vi "TCtrlSeething.vi"() -> ()   [LabVIEW 2018]
uses:
  <vilib>/Utility/miscctls.llb/LVPointTypeDef.ctl
  <vilib>/Utility/error.llb/DialogType.ctl
panel:
  in  "基数可见":bool
  in  "增量可见":bool
  in  "标题可见":bool
  in  "标签可见":bool
  in  "数字精度":i32 min=0 max=8 step=1
  in  "显示格式":u16(ring) items=["十进制", "科学计数法", "工程计数", "二进制", "八进制", "十六进制", "相对时间", "时间和日期", "SI符号"]
  in  "字体格式":enum16{"正常", "粗体", "斜体", "删除线", "下划线"}(ring)
  in  "字体大小":i32
  in  "文本文字颜色":u32(colorbox)
  in  "文本前景色":u32(colorbox)
  in  "文本背景色":u32(colorbox)
  in  "控件前景色":u32(colorbox)
  in  "控件背景色":u32(colorbox)
  in  "数值":dbl
  in  "控件排布前面板.位置_前.位置":T1 caption="数字显示控件大小"
  in  "设定":bool
  out "Error Report":string
  out "Current State":string
  in  "Data Structure":T2
  in  "OK":bool
  in  "Exit Program":bool
  in  "Error":bool
  in  "Parameter":T3={"Q-HighLevel"="Q-HighLevel", "Q-Local"="Enginex", "Data"=variant}
  # "字体设置"
  # "示例"
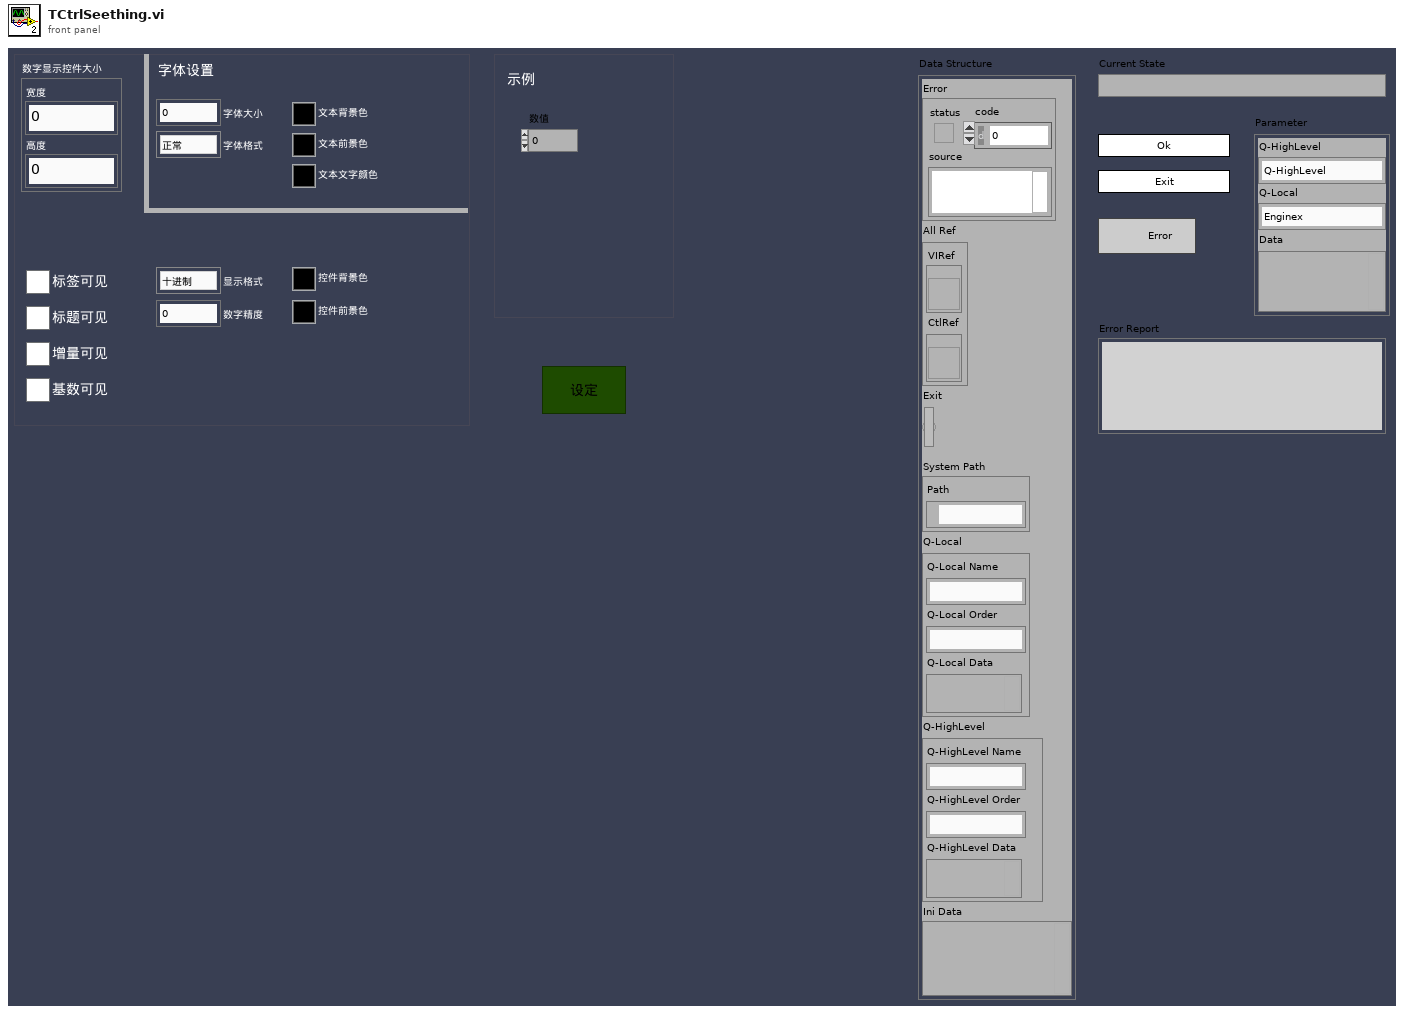
[diagram p1: front panel]
types:
  T1 = typedef "LVPointTypeDef.ctl" = cluster{"Horizontal":i16, "Vertical":i16}
  T2 = cluster{"Error":errorcluster, "All Ref":cluster{"VIRef":refnum<vi>, "CtlRef":refnum<vi>}, "Exit":bool, "System Path":cluster{"Path":path}, "Q-Local":cluster{"Q-Local Name":string, "Q-Local Order":string, "Q-Local Data":variant}, "Q-HighLevel":cluster{"Q-HighLevel Name":string, "Q-HighLevel Order":string, "Q-HighLevel Data":variant}, "Ini Data":variant}
  T3 = cluster{"Q-HighLevel":string, "Q-Local":string, "Data":variant}
  T4 = typedef "eventvkey.ctl" = enum16{"ASCII", "Enter", "Return", "Shift", "Ctrl", "Alt", "Cmd", "Opt", "Caps", "NumLock", "Clear", "Break", "Up", "Down", "Left", "Right", "Insert", "Delete", "Home", "End", "PageUp", "PageDown", "Escape", "Help", "Pause", "ScrollLock", "F1", "F2", "F3", "F4", "F5", "F6", "F7", "F8", "F9", "F10", "F11", "F12", "F13", "F14", "F15", "F16", "F17", "F18", "F19", "F20", "F21", "F22", "F23", "F24", "Play", "VolumeUp", "VolumeDown", "Mute", "Two Byte Char"}
  T5 = typedef "DialogType.ctl" = u16
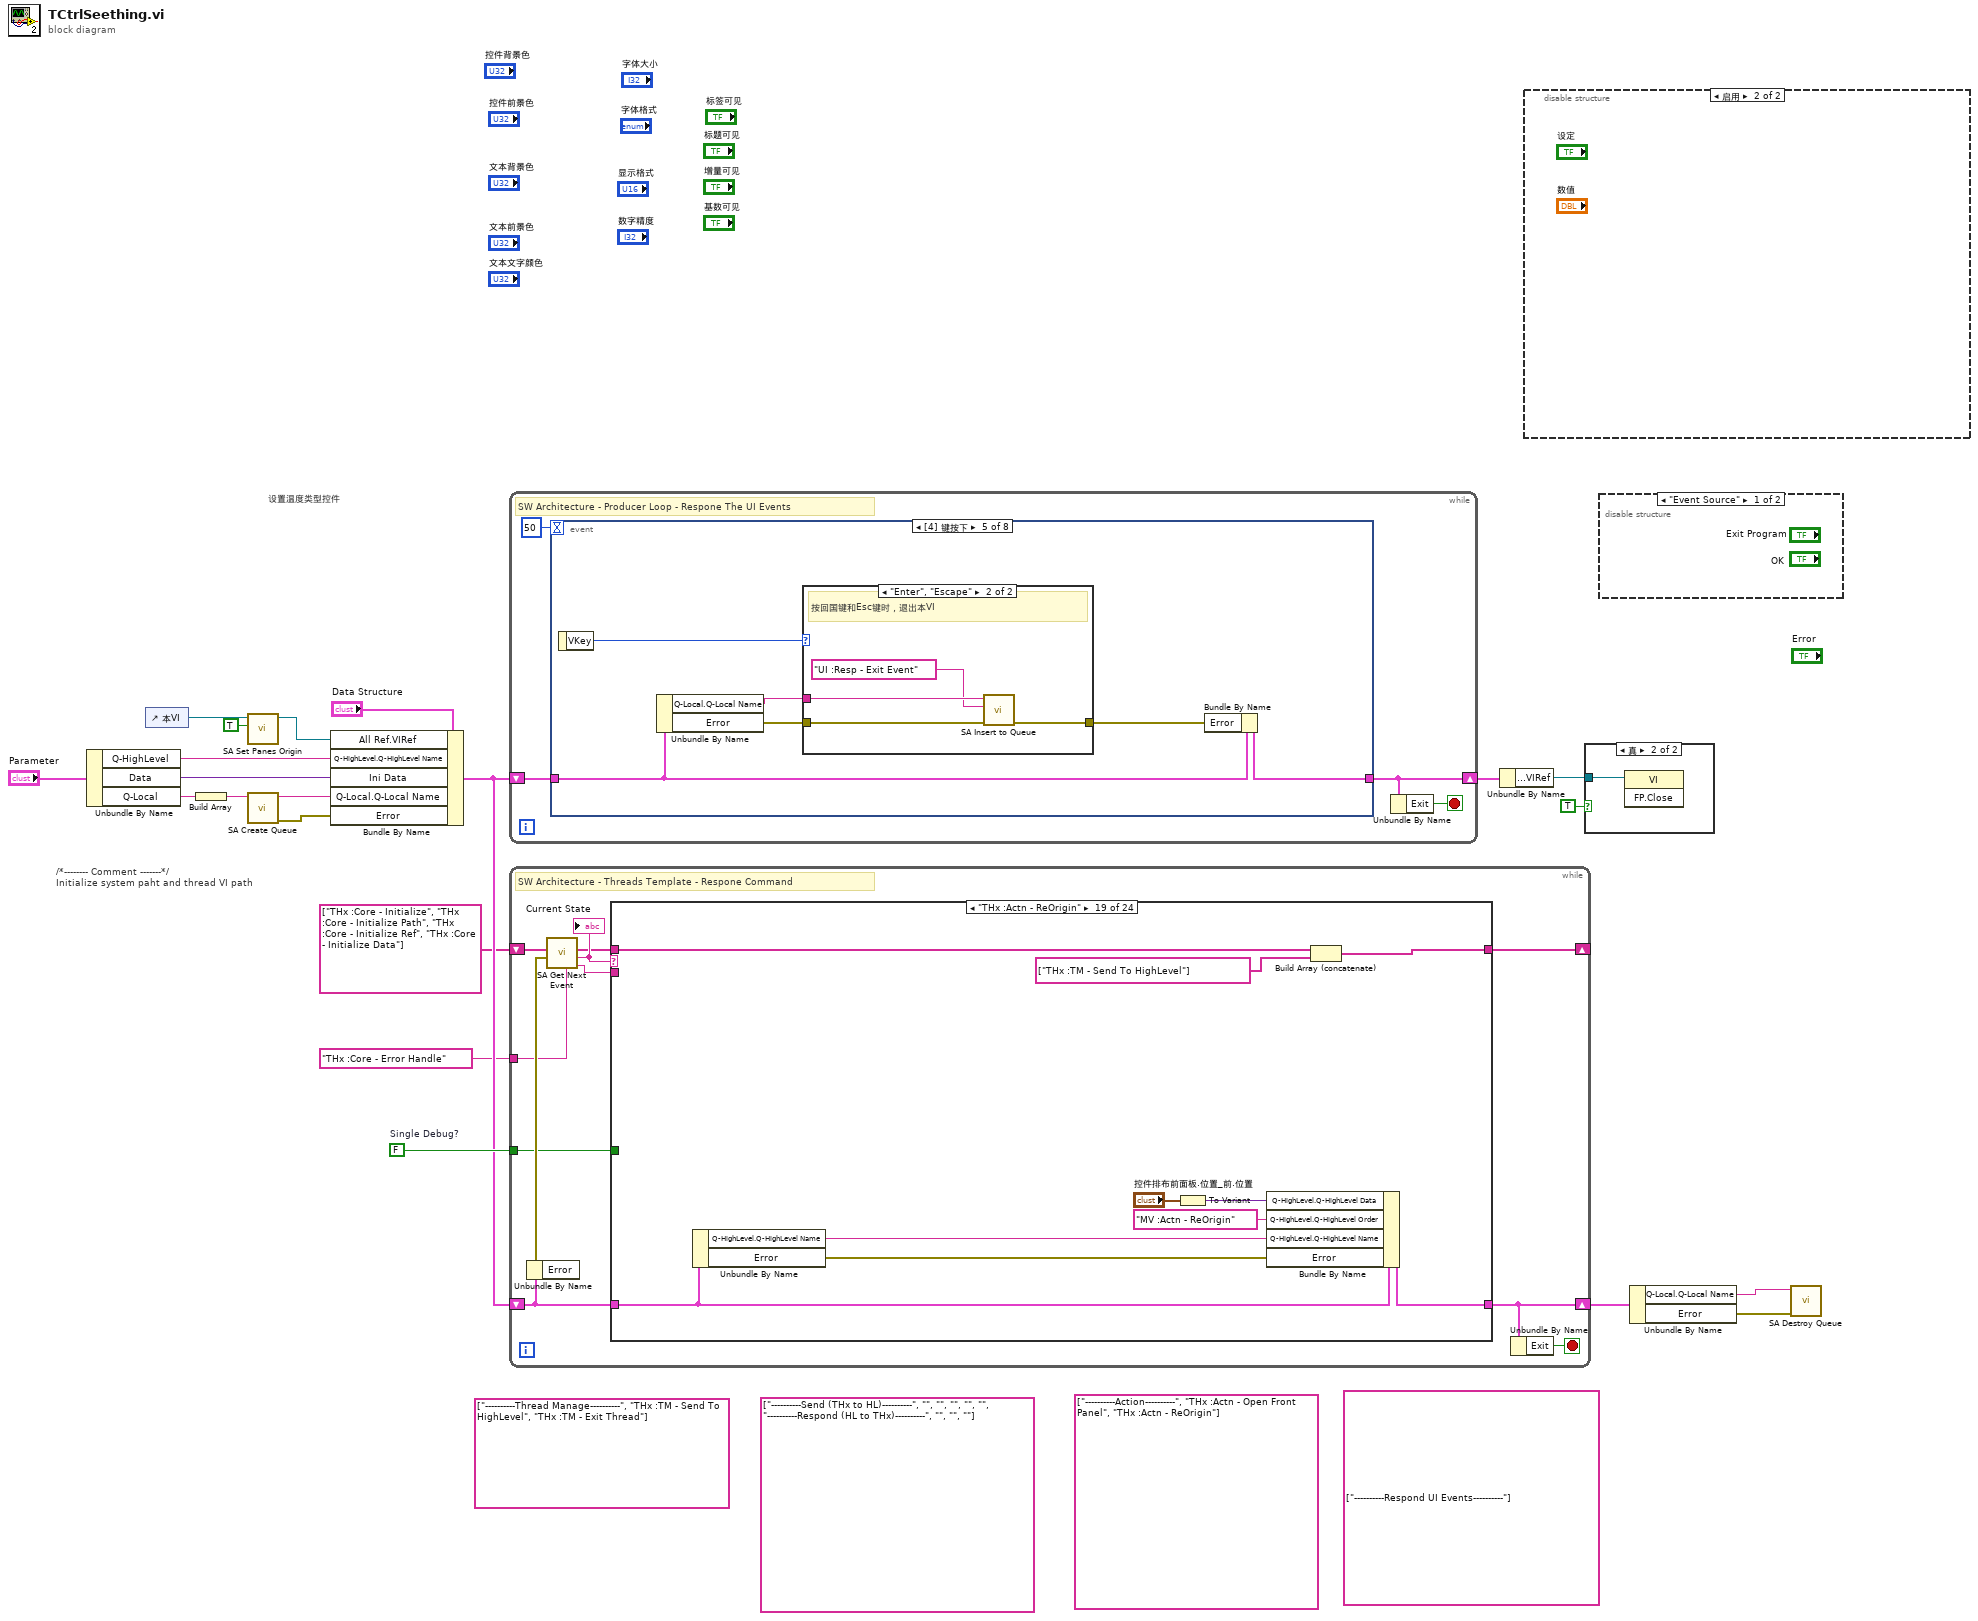
[diagram p0: block diagram]
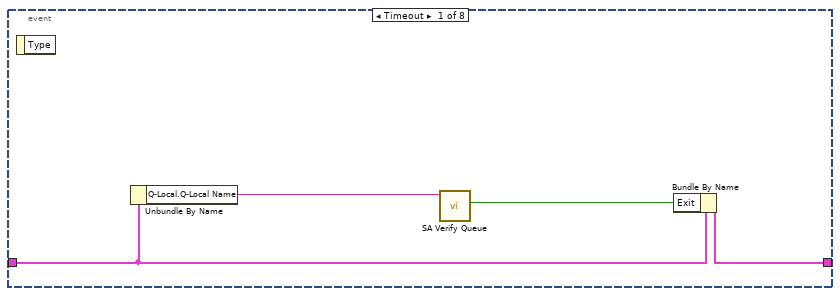
[diagram p5: hidden frame]
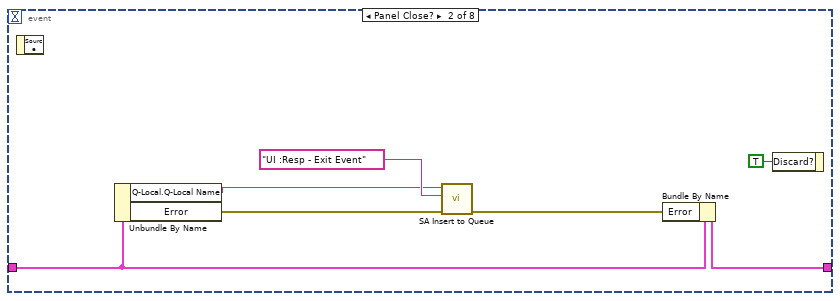
[diagram p6: hidden frame]
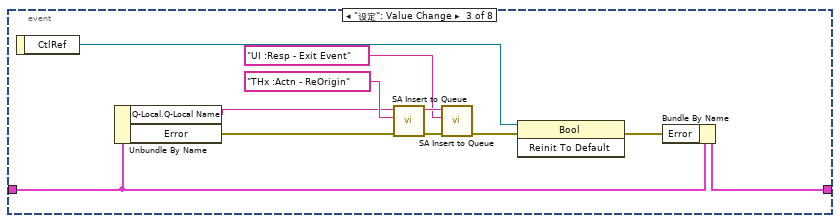
[diagram p7: hidden frame]
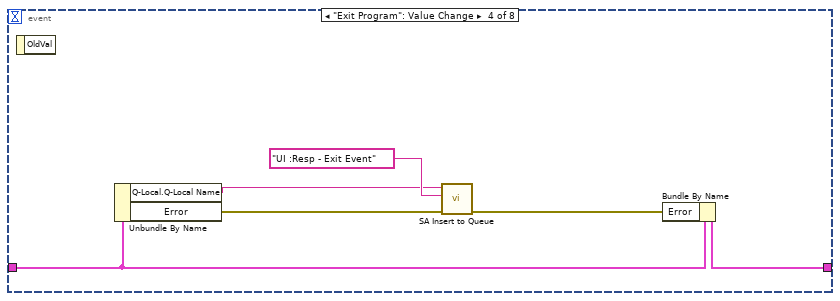
[diagram p8: hidden frame]
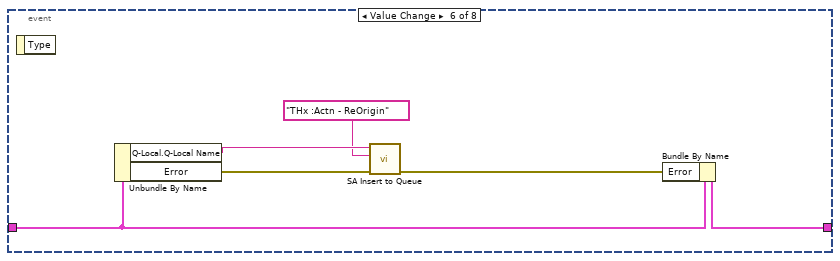
[diagram p10: hidden frame]
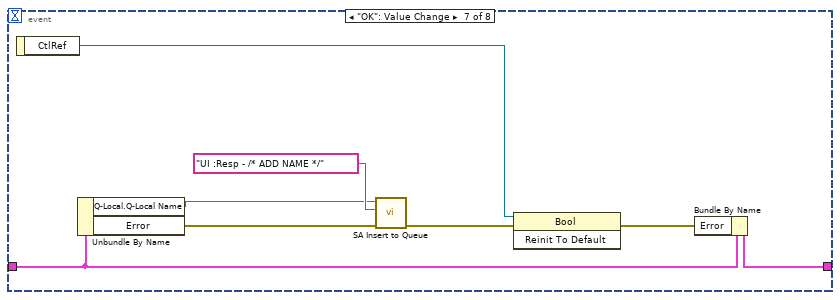
[diagram p11: hidden frame]
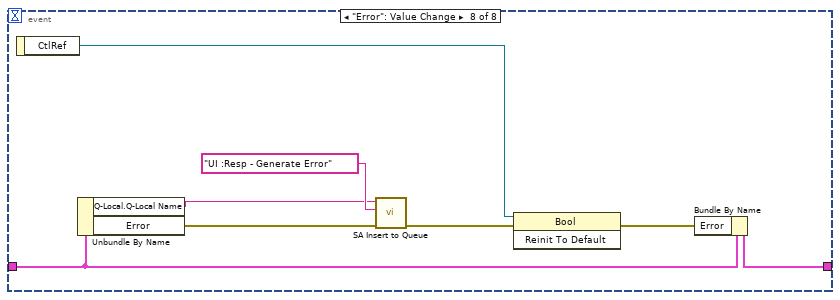
[diagram p12: hidden frame]
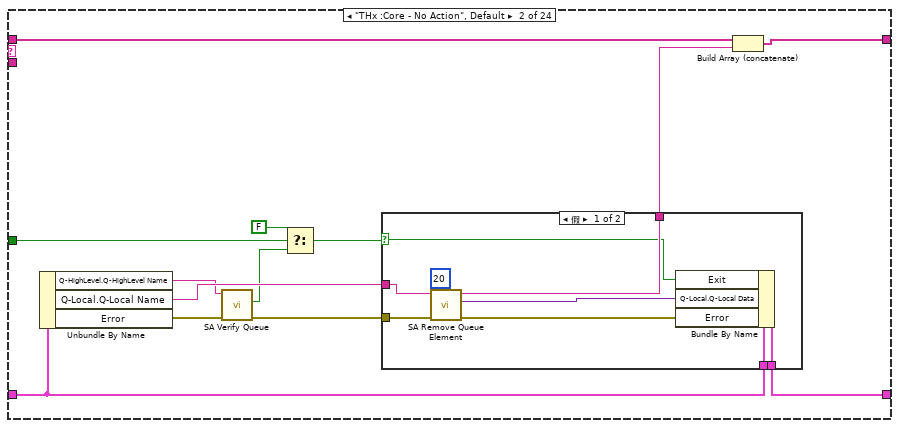
[diagram p14: hidden frame]
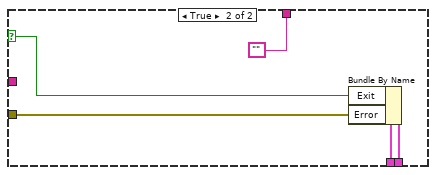
[diagram p15: hidden frame]
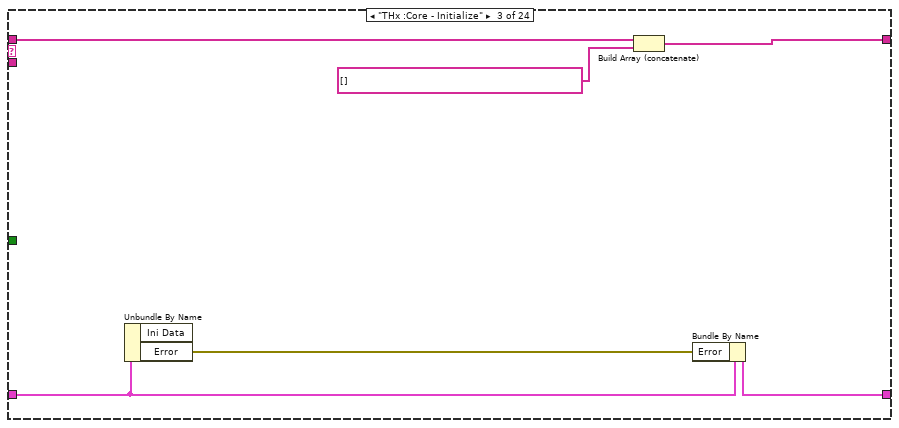
[diagram p16: hidden frame]
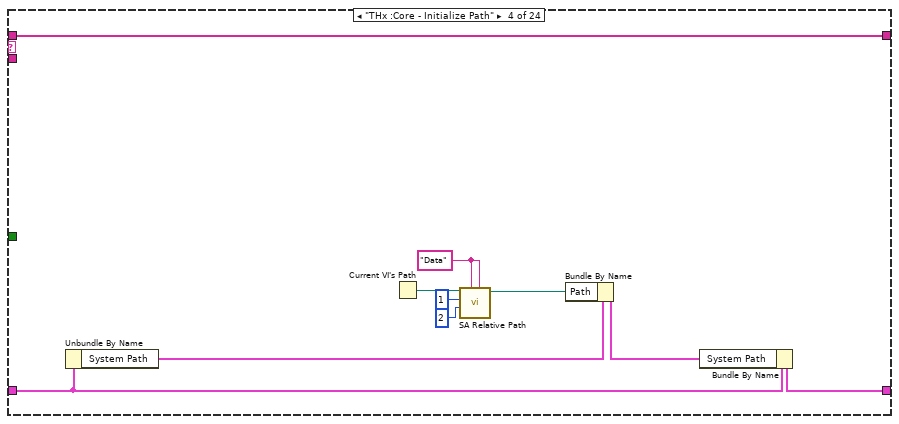
[diagram p17: hidden frame]
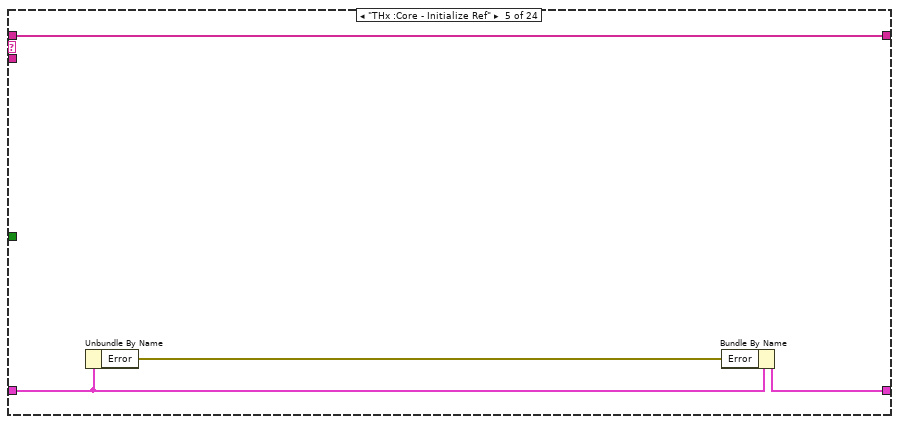
[diagram p18: hidden frame]
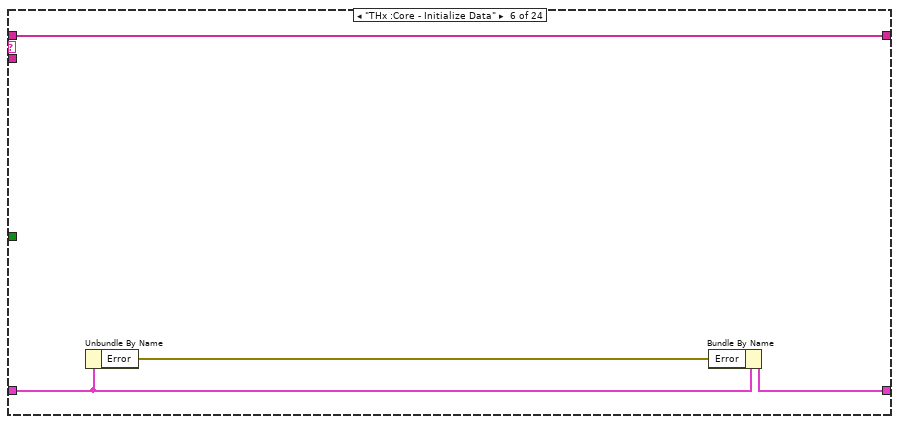
[diagram p19: hidden frame]
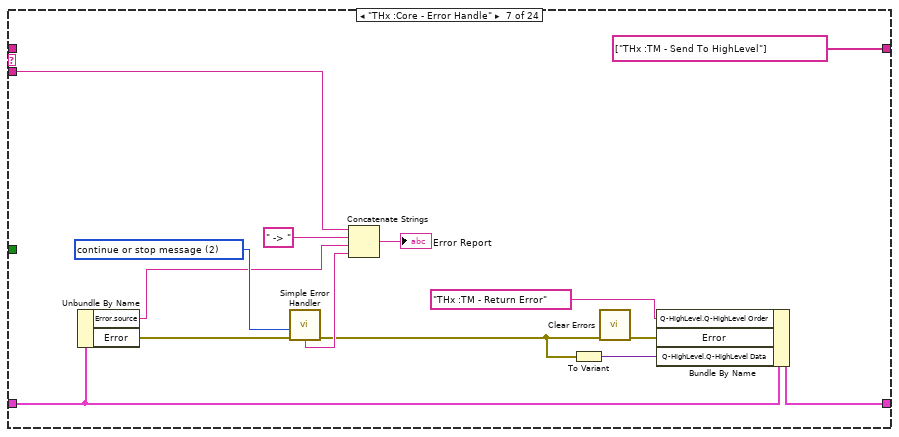
[diagram p20: hidden frame]
diagram:
  w16 = FALSE  # Single Debug?
  (unwired) string[] ["----------Action----------", "THx :Actn - Open Front Panel", "THx :Actn - ReOrigin"]
  (unwired) string[] ["----------Respond UI Events----------"]
  (unwired) string[] ["----------Send (THx to HL)----------", "", "", "", "", "", "----------Respond (HL to THx)----------", "", "", ""]
  (unwired) string[] ["----------Thread Manage----------", "THx :TM - Send To HighLevel", "THx :TM - Exit Thread"]
  # "设置温度类型控件"
  # "/*-------- Comment -------*/\nInitialize system paht and thread VI path"
  n1 = Unbundle By Name("Parameter") -> ("Q-HighLevel"=w15:string, "Data"=w17:variant, "Q-Local"=w14:string)
  n2 = control-ref of="本VI"() -> (w18:refnum<vi>)
  n3 = Build Array(w14) -> (w12:string[])
  n4 = call <vilib>:"SA Set Panes Origin.vi"("Enable? (F)"=TRUE, "VI Ref in"=w18) -> ("VI Ref out"=w19:refnum<vi>)  [unwired: 9 in]
  n5 = call <vilib>:"SA Create Queue.vi"("Queue Name"=w12) -> ("error out"=w7:errorcluster)  [unwired: 10 in]
  n6 = Bundle By Name(cluster="Data Structure", "All Ref.VIRef"=w19, "Q-HighLevel.Q-HighLevel Name"=w15, "Ini Data"=w17, "Q-Local.Q-Local Name"=w14, "Error"=w7) -> (w8:T2)
  n7 = while {
    shift-right: [w22] -> w9
    shift-left: w8 -> [w23]
    stop <- w21 stop-if-true
    # "SW Architecture - Producer Loop - Respone The UI Events"
    n8 = event shown="[4] 键按下" {
      selector: _ -> [_ _ _ _ _ _ _ _]
      dyn-events: _ -> [_ _ _ _ _ _ _ _]
      timeout: 50 -> [_ _ _ _ _ _ _ _]
      tunnel: w23 -> [w26 w33 w43 w49 w56 w67 w71 w79]
      tunnel: [w28 w32 w42 w48 w55 w66 w70 w78] -> w22
      event Timeout {
        n9 = event-data() -> ()  [unwired: 1 in, 1 out]
        n10 = Unbundle By Name(w26) -> ("Q-Local.Q-Local Name"=w25:string)
        n11 = call <vilib>:"SA Verify Queue.vi"("Queue Name in"=w25) -> ("Not A Queue?"=w27:bool)  [unwired: 6 in, 3 out]
        n12 = Bundle By Name(cluster=w26, "Exit"=w27) -> (w28:T2)
      }
      event Panel Close? {
        n13 = event-data() -> ()  [unwired: 1 in, 1 out]
        n14 = Unbundle By Name(w33) -> ("Q-Local.Q-Local Name"=w30:string, "Error"=w34:errorcluster)
        n15 = call <vilib>:"SA Insert to Queue.vi"("error in"=w34, "Event"="UI :Resp - Exit Event", "Queue Name"=w30) -> ("error out"=w31:errorcluster)  [unwired: 8 in]
        n16 = Bundle By Name(cluster=w33, "Error"=w31) -> (w32:T2)
        n17 = event-data("Discard?"=TRUE ("放弃？")) -> ()  [unwired: 1 in, 1 out]
      }
      event "设定": Value Change {
        n18 = event-data() -> ("CtlRef"=w40:refnum<vi>)  [unwired: 1 in]
        n19 = Unbundle By Name(w43) -> ("Q-Local.Q-Local Name"=w37:string, "Error"=w44:errorcluster)
        n20 = call <vilib>:"SA Insert to Queue.vi"("error in"=w44, "Event"="THx :Actn - ReOrigin", "Queue Name"=w37) -> ("error out"=w39:errorcluster)  [unwired: 8 in]
        n21 = call <vilib>:"SA Insert to Queue.vi"("error in"=w39, "Event"="UI :Resp - Exit Event", "Queue Name"=w37) -> ("error out"=w38:errorcluster)  [unwired: 8 in]
        n22 = invoke class="Bool" method="Reinit To Default"(reference=w40, error in=w38) -> (error out=w41:errorcluster)  [unwired: 1 in, 2 out]
        n23 = Bundle By Name(cluster=w43, "Error"=w41) -> (w42:T2)
      }
      event "Exit Program": Value Change {
        n24 = event-data() -> ()  [unwired: 1 in, 1 out]
        n25 = Unbundle By Name(w49) -> ("Q-Local.Q-Local Name"=w46:string, "Error"=w50:errorcluster)
        n26 = call <vilib>:"SA Insert to Queue.vi"("error in"=w50, "Event"="UI :Resp - Exit Event", "Queue Name"=w46) -> ("error out"=w47:errorcluster)  [unwired: 8 in]
        n27 = Bundle By Name(cluster=w49, "Error"=w47) -> (w48:T2)
      }
      event Key Down {
        n28 = event-data() -> ("VKey"=w52:T4)  [unwired: 1 in]
        n29 = Unbundle By Name(w56) -> ("Q-Local.Q-Local Name"=w53:string, "Error"=w57:errorcluster)
        n30 = case shown="\"Enter\", \"Escape\"" w52 {
          tunnel: w57 -> [w58 w62]
          tunnel: [w58 w61] -> w54
          tunnel: w53 -> [_ w60]
          frame "ASCII", Default {
          }
          frame "Enter", "Escape" {
            # "按回国键和Esc键时，退出本VI"
            n31 = call <vilib>:"SA Insert to Queue.vi"("error in"=w62, "Event"="UI :Resp - Exit Event", "Queue Name"=w60) -> ("error out"=w61:errorcluster)  [unwired: 8 in]
          }
        }
        n32 = Bundle By Name(cluster=w56, "Error"=w54) -> (w55:T2)
      }
      event Value Change {
        n33 = event-data() -> ()  [unwired: 1 in, 1 out]
        n34 = Unbundle By Name(w67) -> ("Q-Local.Q-Local Name"=w65:string, "Error"=w68:errorcluster)
        n35 = call <vilib>:"SA Insert to Queue.vi"("error in"=w68, "Event"="THx :Actn - ReOrigin", "Queue Name"=w65) -> ("error out"=w63:errorcluster)  [unwired: 8 in]
        n36 = Bundle By Name(cluster=w67, "Error"=w63) -> (w66:T2)
      }
      event "OK": Value Change {
        n37 = event-data() -> ("CtlRef"=w76:refnum<vi>)  [unwired: 1 in]
        n38 = Unbundle By Name(w71) -> ("Q-Local.Q-Local Name"=w69:string, "Error"=w74:errorcluster)
        n39 = call <vilib>:"SA Insert to Queue.vi"("error in"=w74, "Event"="UI :Resp - /* ADD NAME */", "Queue Name"=w69) -> ("error out"=w73:errorcluster)  [unwired: 8 in]
        n40 = invoke class="Bool" method="Reinit To Default"(reference=w76, error in=w73) -> (error out=w72:errorcluster)  [unwired: 1 in, 2 out]
        n41 = Bundle By Name(cluster=w71, "Error"=w72) -> (w70:T2)
      }
      event "Error": Value Change {
        n42 = event-data() -> ("CtlRef"=w84:refnum<vi>)  [unwired: 1 in]
        n43 = Unbundle By Name(w79) -> ("Q-Local.Q-Local Name"=w77:string, "Error"=w82:errorcluster)
        n44 = call <vilib>:"SA Insert to Queue.vi"("error in"=w82, "Event"="UI :Resp - Generate Error", "Queue Name"=w77) -> ("error out"=w81:errorcluster)  [unwired: 8 in]
        n45 = invoke class="Bool" method="Reinit To Default"(reference=w84, error in=w81) -> (error out=w80:errorcluster)  [unwired: 1 in, 2 out]
        n46 = Bundle By Name(cluster=w79, "Error"=w80) -> (w78:T2)
      }
    }
    n47 = Unbundle By Name(w22) -> ("Exit"=w21:bool)
  }
  n48 = while {
    shift-right: [w89] -> w6
    shift-left: w8 -> [w91]
    shift-right: [w92] -> _
    shift-left: string[] ["THx :Core - Initialize", "THx :Core - Initialize Path", "THx :Core - Initialize Ref", "THx :Core - Initialize Data"] -> [w95]
    tunnel: "THx :Core - Error Handle" ("Error Handle") -> [w87]
    tunnel: w16 -> [w85]
    stop <- w88 stop-if-true
    # "SW Architecture - Threads Template - Respone Command"
    n49 = Unbundle By Name(w91) -> ("Error"=w90:errorcluster)
    n50 = call <vilib>:"SA Get Next Event.vi"("Error Handle"=w87, "error in"=w90, "event queue in"=w95) -> ("prev event"=w86:string, "next event"=w94:string, "event queue out"=w93:string[])  [unwired: 6 in]
    "Current State" <- w94
    n51 = case shown="\"THx :Actn - ReOrigin\"" w94 {
      tunnel: w91 -> [w96 w110 w128 w138 w142 w146 w161 w164 w168 w175 w189 w195 w200 w202 w207 w213 w215 w220 w230 w236 w238 w243 w249 w254]
      tunnel: w93 -> [w97 w108 w130 w140 w144 w148 _ w167 w169 w178 w194 w196 w201 w203 w208 w211 w216 w221 w231 w237 w239 w241 w247 w252]
      tunnel: [w97 w107 w129 w140 w144 w148 string[] ["THx :TM - Send To HighLevel"] w167 w169 w178 w193 w196 w197 w203 w204 w210 w216 w217 w227 w237 w239 w240 w246 w251] -> w92
      tunnel: [w96 w109 w127 w139 w143 w147 w162 w165 w168 w174 w191 w195 w198 w202 w205 w212 w215 w219 w229 w235 w238 w242 w248 w253] -> w89
      tunnel: w86 -> [_ _ _ _ _ _ w157 _ _ _ _ _ _ _ _ _ _ _ _ _ _ _ _ _]
      tunnel: w85 -> [_ w102 _ _ _ _ _ _ _ _ _ _ _ _ _ _ _ _ _ _ _ _ _ _]
      frame "----------Core Status----------" {
      }
      frame "THx :Core - No Action", Default {
        n52 = Unbundle By Name(w110) -> ("Q-HighLevel.Q-HighLevel Name"=w99:string, "Q-Local.Q-Local Name"=w105:string, "Error"=w104:errorcluster)
        n53 = call <vilib>:"SA Verify Queue.vi"("error in"=w104, "Queue Name in"=w99) -> ("error out"=w103:errorcluster, "Not A Queue?"=w98:bool)  [unwired: 5 in, 2 out]
        n54 = Select(t=FALSE, s=w102, f=w98) -> (s? t:f=w100:bool)
        n55 = case shown="假" w100 {
          selector: w100 -> [w111 w122]
          tunnel: w110 -> [w117 w123]
          tunnel: [w116 w120] -> w109
          tunnel: [w115 "" ("Event")] -> w106
          tunnel: w105 -> [w113 _]
          tunnel: w103 -> [w112 w121]
          frame False {
            n56 = call <vilib>:"SA Remove Queue Element.vi"("Time out (10)"=20 ("Time out(-1)_queue out"), "error in"=w112, "Queue Name"=w113) -> ("error out"=w119:errorcluster, "Data"=w118:variant, "Event"=w115:string)  [unwired: 5 in, 1 out]
            n57 = Bundle By Name(cluster=w117, "Exit"=w111, "Q-Local.Q-Local Data"=w118, "Error"=w119) -> (w116:T2)
          }
          frame True {
            n58 = Bundle By Name(cluster=w123, "Exit"=w122, "Error"=w121) -> (w120:T2)
          }
        }
        n59 = Build Array (concatenate)(w108, w106) -> (w107:string[])
      }
      frame "THx :Core - Initialize" {
        n60 = Unbundle By Name(w128) -> ("Error"=w126:errorcluster)  [unwired: 1 out]
        n61 = Build Array (concatenate)(w130, string[] [] ("数组")) -> (w129:string[])
        n62 = Bundle By Name(cluster=w128, "Error"=w126) -> (w127:T2)
      }
      frame "THx :Core - Initialize Path" {
        w133 = "Data" ("Data Folder Path")
        n63 = Unbundle By Name(w138) -> ("System Path"=w132:cluster{"Path":path})
        n64 = Current VI's Path() -> (path=w134:path)
        n65 = call <vilib>:"SA Relative Path.vi"("Development Relative Path"=w133, "Run Time Relative path"=w133, "Run-Time File Depth"=2, "Development File Depth"=1, "Root Path"=w134) -> ("Relative Path"=w137:path)  [unwired: 5 in, 1 out]
        n66 = Bundle By Name(cluster=w132, "Path"=w137) -> (w131:cluster{"Path":path})
        n67 = Bundle By Name(cluster=w138, "System Path"=w131) -> (w139:T2)
      }
      frame "THx :Core - Initialize Ref" {
        n68 = Unbundle By Name(w142) -> ("Error"=w141:errorcluster)
        n69 = Bundle By Name(cluster=w142, "Error"=w141) -> (w143:T2)
      }
      frame "THx :Core - Initialize Data" {
        n70 = Unbundle By Name(w146) -> ("Error"=w145:errorcluster)
        n71 = Bundle By Name(cluster=w146, "Error"=w145) -> (w147:T2)
      }
      frame "THx :Core - Error Handle" {
        w158 = T5 2 items=["no dialog", "OK message", "continue or stop message", "OK message + warnings", "continue/stop + warnings"] ("type of dialog (OK msg:1)")
        n72 = Unbundle By Name(w161) -> ("Error.source"=w155:string, "Error"=w159:errorcluster)
        n73 = call <vilib>:"Simple Error Handler.vi"("type of dialog (OK msg:1)"=w158, "error in (no error)"=w159) -> ("error out"=w151:errorcluster, "message"=w154:string)  [unwired: 3 in, 3 out]
        n74 = Concatenate Strings(w157, " -> " ("字符串"), w155, w154) -> (→"Error Report":string)
        n75 = To Variant(anything=w151) -> (Variant=w150:variant)
        n76 = call <vilib>:"Clear Errors.vi"("error in (no error)"=w151) -> ("error out"=w160:errorcluster)  [unwired: 5 in, 1 out]
        n77 = Bundle By Name(cluster=w161, "Q-HighLevel.Q-HighLevel Order"="THx :TM - Return Error" ("Q-Local.Q-Local Order"), "Error"=w160, "Q-HighLevel.Q-HighLevel Data"=w150) -> (w162:T2)
      }
      frame "THx :Core - Exit Thread" {
        n78 = Unbundle By Name(w164) -> ("Error"=w166:errorcluster)
        n79 = Bundle By Name(cluster=w164, "Exit"=TRUE, "Error"=w166) -> (w165:T2)
      }
      frame "----------Thread Manage----------" {
      }
      frame "THx :TM - Send To HighLevel" {
        n80 = Unbundle By Name(w175) -> ("Q-HighLevel.Q-HighLevel Name"=w177:string, "Q-HighLevel.Q-HighLevel Order"=w172:string, "Q-HighLevel.Q-HighLevel Data"=w171:variant, "Error"=w176:errorcluster)
        n81 = call <vilib>:"SA Verify Queue.vi"("Queue Name in"=w177) -> ("Not A Queue?"=w173:bool)  [unwired: 6 in, 3 out]
        n82 = case shown="假" w173 {
          tunnel: w176 -> [w184 w185]
          tunnel: w177 -> [w183 _]
          tunnel: w172 -> [w181 _]
          tunnel: w171 -> [w182 _]
          tunnel: [w180 w185] -> w170
          frame False {
            n83 = call <vilib>:"SA Insert to Queue.vi"("Time out (10)"=50 ("Time out(-1)_queue in"), "error in"=w184, "Data"=w182, "Event"=w181, "Queue Name"=w183) -> ("error out"=w180:errorcluster)  [unwired: 6 in]
          }
          frame True {
          }
        }
        n84 = Bundle By Name(cluster=w175, "Error"=w170) -> (w174:T2)
      }
      frame "THx :TM - Exit Thread" {
        n85 = Unbundle By Name(w189) -> ("Q-Local.Q-Local Name"=w188:string, "Error"=w186:errorcluster)
        n86 = To Variant(anything=w188) -> (Variant=w187:variant)
        n87 = Bundle By Name(cluster=w189, "Q-HighLevel.Q-HighLevel Order"="THx :TM - Delete Dynamic Thread", "Q-HighLevel.Q-HighLevel Data"=w187, "Error"=w186) -> (w191:T2)
        n88 = Build Array (concatenate)(w194, string[] ["THx :TM - Send To HighLevel", "THx :Core - Exit Thread"] ("数组")) -> (w193:string[])
      }
      frame "----------Send (THx to HL)----------" {
      }
      frame "THx :HL - /* ADD NAME */" {
        n89 = Unbundle By Name(w200) -> ("Error"=w199:errorcluster)
        n90 = Build Array (concatenate)(w201) -> (w197:string[])
        n91 = Bundle By Name(cluster=w200, "Error"=w199) -> (w198:T2)
      }
      frame "----------Respond (HL to THx)----------" {
      }
      frame "HL :THx - /* ADD NAME */" {
        n92 = Unbundle By Name(w207) -> ("Error"=w206:errorcluster)
        n93 = Build Array (concatenate)(w208) -> (w204:string[])
        n94 = Bundle By Name(cluster=w207, "Error"=w206) -> (w205:T2)
      }
      frame "TM :THx - Quit Dynamic Thread" {
        n95 = Unbundle By Name(w213) -> ("Error"=w214:errorcluster)
        n96 = Bundle By Name(cluster=w213, "Error"=w214) -> (w212:T2)
        n97 = Build Array (concatenate)(w211, string[] ["THx :TM - Exit Thread"] ("数组")) -> (w210:string[])
      }
      frame "----------Actions----------" {
      }
      frame "THx :Actn - /* ADD NAME */" {
        n98 = Unbundle By Name(w220) -> ("Error"=w218:errorcluster)
        n99 = Build Array (concatenate)(w221) -> (w217:string[])
        n100 = Bundle By Name(cluster=w220, "Error"=w218) -> (w219:T2)
      }
      frame "THx :Actn - ReOrigin" {
        n101 = Unbundle By Name(w230) -> ("Q-HighLevel.Q-HighLevel Name"=w226:string, "Error"=w228:errorcluster)
        n102 = To Variant(anything="控件排布前面板.位置_前.位置") -> (Variant=w224:variant)
        n103 = Bundle By Name(cluster=w230, "Q-HighLevel.Q-HighLevel Data"=w224, "Q-HighLevel.Q-HighLevel Order"="MV :Actn - ReOrigin", "Q-HighLevel.Q-HighLevel Name"=w226, "Error"=w228) -> (w229:T2)
        n104 = Build Array (concatenate)(w231, string[] ["THx :TM - Send To HighLevel"] ("数组")) -> (w227:string[])
      }
      frame "THx :Actn - Open Front Panel" {
        n105 = Unbundle By Name(w236) -> ("All Ref.VIRef"=w232:refnum<vi>, "Error"=w234:errorcluster)
        n106 = invoke class="VI" method="FP.Open"(reference=w232, error in=w234) -> (error out=w233:errorcluster)  [unwired: 3 in, 4 out]
        n107 = Bundle By Name(cluster=w236, "Error"=w233) -> (w235:T2)
      }
      frame "----------Respond Events----------" {
      }
      frame "UI :Resp - /* ADD NAME */" {
        n108 = Unbundle By Name(w243) -> ("Error"=w244:errorcluster)
        n109 = Build Array (concatenate)(w241) -> (w240:string[])
        n110 = Bundle By Name(cluster=w243, "Error"=w244) -> (w242:T2)
      }
      frame "UI :Resp - Generate Error" {
        n111 = Unbundle By Name(w249) -> ()  [unwired: 1 out]
        n112 = Build Array (concatenate)(w247) -> (w246:string[])
        n113 = Bundle By Name(cluster=w249, "Error"=errorcluster {"status"=TRUE, "code"=-1, "source"="Error Test"}) -> (w248:T2)
      }
      frame "UI :Resp - Exit Event" {
        n114 = Unbundle By Name(w254) -> ("Error"=w255:errorcluster)
        n115 = Build Array (concatenate)(w252, string[] ["THx :TM - Exit Thread"] ("数组")) -> (w251:string[])
        n116 = Bundle By Name(cluster=w254, "Error"=w255) -> (w253:T2)
      }
    }
    n117 = Unbundle By Name(w89) -> ("Exit"=w88:bool)
  }
  n118 = Unbundle By Name(w9) -> ("All Ref.VIRef"=w10:refnum<vi>)
  n119 = disable-structure shown="启用" {
    frame Disabled {
    }
    frame Enabled {
    }
  }
  n120 = case shown="真" TRUE {
    tunnel: w10 -> [_ w256]
    frame False {
    }
    frame True {
      n121 = invoke class="VI" method="FP.Close"(reference=w256) -> ()  [unwired: 2 in, 3 out]
    }
  }
  n122 = disable-structure shown="\"Event Source\"" {
    frame condition #0 (active) {
    }
    frame condition #1 {
    }
  }
  n123 = Unbundle By Name(w6) -> ("Q-Local.Q-Local Name"=w4:string, "Error"=w5:errorcluster)
  n124 = call <vilib>:"SA Destroy Queue.vi"("error in"=w5, "Queue Name"=w4) -> ()  [unwired: 9 in, 1 out]
